vi "Play.vi"() -> ()   [LabVIEW 2019]
uses:
  System.Data.SQLite
  HeirDAL Library/Models Library/Object Class/Object.lvclass
  HeirDAL Library/Models Library/Attribute Class/Attribute.lvclass
  <vilib>/addons/h5labview2/dataset/H5D.lvlib
panel:
  out "ConnectionString":string
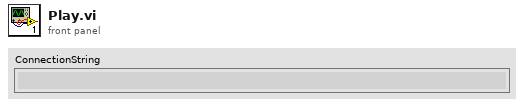
[diagram p1: front panel]
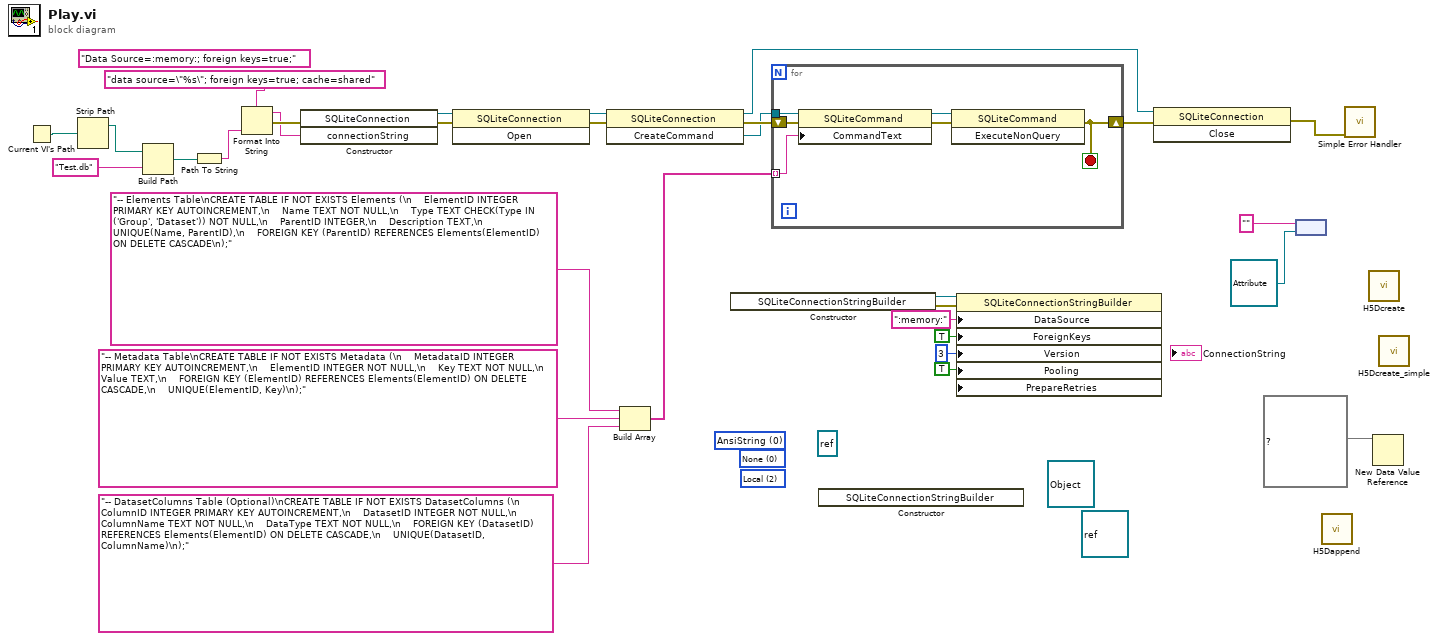
[diagram p0: block diagram]
diagram:
  (unwired) refnum<class> refnum ("LabVIEW Object")
  (unwired) refnum<class "Object.lvclass"> refnum ("HierDAL Library.lvlib:Models.lvlib:Object.lvclass")
  (unwired) refnum<k24> refnum ("new reference")
  (unwired) 2 items=["Unspecified", "Utc", "Local"] ("DateTimeKind")
  (unwired) 0 items=["AnsiString"=0, "Binary"=1, "Byte"=2, "Boolean"=3, "Currency"=4, "Date"=5, "DateTime"=6, "Decimal"=7, "Double"=8, "Guid"=9, "Int16"=10, "Int32"=11, "Int64"=12, "Object"=13, "SByte"=14, "Single"=15, "String"=16, "Time"=17, "UInt16"=18, "UInt32"=19, "UInt64"=20, "VarNumeric"=21, "AnsiStringFixedLength"=22, "StringFixedLength"=23, "Xml"=25, "DateTime2"=26, "DateTimeOffset"=27] ("DefaultDbType")
  (unwired) i64 0 items=["None"=0, "LogPrepare"=1, "LogPreBind"=2, "LogBind"=4, "LogCallbackException"=8, "LogBackup"=16, "NoExtensionFunctions"=32, "BindUInt32AsInt64"=64, "BindAllAsText"=128, "GetAllAsText"=256, "BindAndGetAllAsText"=384, "NoLoadExtension"=512, "NoCreateModule"=1024, "NoBindFunctions"=2048, "NoLogModule"=4096, "LogModuleError"=8192, "LogModuleException"=16384, "LogDefault"=16392, "LogAll"=24607, "TraceWarning"=32768, "ConvertInvariantText"=65536, "BindInvariantText"=131072, "BindAndGetAllAsInvariantText"=131456, "ConvertAndBindInvariantText"=196608, "ConvertAndBindAndGetAllAsInvariantText"=196992, "NoConnectionPool"=262144, "UseConnectionPool"=524288, "UseConnectionTypes"=1048576, "NoGlobalTypes"=2097152, "StickyHasRows"=4194304, "StrictEnlistment"=8388608, "MapIsolationLevels"=16777216, "DetectTextAffinity"=33554432, "DetectStringType"=67108864, "NoConvertSettings"=134217728, "BindDateTimeWithKind"=268435456, "RollbackOnException"=536870912, "DenyOnException"=1073741824, "InterruptOnException"=2147483648, "UnbindFunctionsOnClose"=4294967296, "NoVerifyTextAffinity"=8589934592, "UseConnectionBindValueCallbacks"=17179869184, "UseConnectionReadValueCallbacks"=34359738368, "UseConnectionAllValueCallbacks"=51539607552, "UseParameterNameForTypeName"=68719476736, "UseParameterDbTypeForTypeName"=137438953472, "UseParameterAnythingForTypeName"=206158430208, "NoVerifyTypeAffinity"=274877906944, "AllowNestedTransactions"=549755813888, "BindDecimalAsText"=1099511627776, "GetDecimalAsText"=2199023255552, "BindInvariantDecimal"=4398046511104, "GetInvariantDecimal"=8796093022208, "Default"=13194139549704, "DefaultAndLogAll"=13194139557919, "WaitForEnlistmentReset"=17592186044416, "GetInvariantInt64"=35184372088832, "GetInvariantDouble"=70368744177664, "StrictConformance"=140737488355328, "HidePassword"=281474976710656, "NoCoreFunctions"=562949953421312] ("Flags")
  (unwired) "Data Source=:memory:; foreign keys=true;" ("connectionString")
  n1 = Current VI's Path() -> (path=w16:path)
  n2 = Strip Path(path=w16) -> (stripped path=w15:path)  [unwired: 1 out]
  n3 = Build Path(base path=w15, name or relative path="Test.db") -> (appended path=w17:path)
  n4 = Path To String(path=w17) -> (string=w10:string)
  n5 = Format Into String(format string="data source=\"%s\"; foreign keys=true; cache=shared" ("connectionString"), w10) -> (resulting string=w12:string, error out=w14:errorcluster)  [unwired: 2 in]
  n6 = constructor class="SQLiteConnection"(error in=w14, "connectionString"=w12) -> (reference out=w18:refnum<k24>, error out=w19:errorcluster)  [unwired: 2 in, 2 out]
  n7 = invoke class="SQLiteConnection" method="Open"(reference=w18, error in=w19) -> (reference out=w29:refnum<k24>, error out=w30:errorcluster)  [unwired: 1 in, 1 out]
  n8 = invoke class="SQLiteConnection" method="CreateCommand"(reference=w29, error in=w30) -> (reference out=w25:refnum<k24>, error out=w28:errorcluster, "CreateCommand"=w27:refnum<k24>)  [unwired: 1 in]
  n9 = Build Array("-- Elements Table\nCREATE TABLE IF NOT EXISTS Elements (\n    ElementID INTEGER PRIMARY KEY AUTOINCREMENT,\n    Name TEXT NOT NULL,\n    Type TEXT CHECK(Type IN ('Group', 'Dataset')) NOT NULL,\n    ParentID INTEGER,\n    Description TEXT,\n    UNIQUE(Name, ParentID),\n    FOREIGN KEY (ParentID) REFERENCES Elements(ElementID) ON DELETE CASCADE\n);" ("CommandText"), "-- Metadata Table\nCREATE TABLE IF NOT EXISTS Metadata (\n    MetadataID INTEGER PRIMARY KEY AUTOINCREMENT,\n    ElementID INTEGER NOT NULL,\n    Key TEXT NOT NULL,\n    Value TEXT,\n    FOREIGN KEY (ElementID) REFERENCES Elements(ElementID) ON DELETE CASCADE,\n    UNIQUE(ElementID, Key)\n);" ("CommandText"), "-- DatasetColumns Table (Optional)\nCREATE TABLE IF NOT EXISTS DatasetColumns (\n    ColumnID INTEGER PRIMARY KEY AUTOINCREMENT,\n    DatasetID INTEGER NOT NULL,\n    ColumnName TEXT NOT NULL,\n    DataType TEXT NOT NULL,\n    FOREIGN KEY (DatasetID) REFERENCES Elements(ElementID) ON DELETE CASCADE,\n    UNIQUE(DatasetID, ColumnName)\n);" ("CommandText")) -> (w23:string[])
  n10 = constructor class="SQLiteConnectionStringBuilder"() -> (reference out=w8:refnum<k24>, error out=w9:errorcluster)  [unwired: 3 in, 1 out]
  n11 = for {
    tunnel: w27 -> [w35]
    shift-right: [w31] -> w26
    shift-left: w28 -> [w36]
    tunnel: w23 -> [w32] mode=indexing
    stop <- w31 stop-if-true
    n12 = property class="SQLiteCommand"(reference=w35, error in=w36, "CommandText"=w32) -> (reference out=w33:refnum<k24>, error out=w34:errorcluster)
    n13 = invoke class="SQLiteCommand" method="ExecuteNonQuery"(reference=w33, error in=w34) -> (error out=w31:errorcluster)  [unwired: 1 in, 2 out]
  }
  n14 = constructor class="SQLiteConnectionStringBuilder"() -> ()  [unwired: 3 in, 3 out]
  n15 = property class="SQLiteConnectionStringBuilder" props=["DataSource", "ForeignKeys", "Version", "Pooling", "PrepareRetries"](reference=w8, error in=w9, "DataSource"=":memory:", "ForeignKeys"=TRUE, "Version"=3, "Pooling"=TRUE) -> ()  [unwired: 1 in, 2 out]
  n16 = invoke class="SQLiteConnection" method="Close"(reference=w25, error in=w26) -> (error out=w20:errorcluster)  [unwired: 1 in, 2 out]
  n17 = node("", refnum<class "Attribute.lvclass"> refnum ("HierDAL Library.lvlib:Models.lvlib:Attribute.lvclass")) -> ()  [unwired: 1 out]
  n18 = call <vilib>:"H5Dappend.vi"() -> ()  [unwired: 8 in, 4 out]
  n19 = call <vilib>:"Simple Error Handler.vi"("error in (no error)"=w20) -> ()  [unwired: 4 in, 5 out]
  n20 = call <vilib>:"H5Dcreate.vi"() -> ()  [unwired: 8 in, 2 out]
  n21 = New Data Value Reference(data value=map{string, refnum<class "Attribute.lvclass">} {} ("map")) -> ()  [unwired: 1 in, 2 out]
  n22 = call <vilib>:"H5Dcreate_simple.vi"() -> ()  [unwired: 10 in, 2 out]
